vi "Save Recall List Program.vi"(8 "error in (no error)":errorcluster, 9 "List Number (1)":u32=1 min=1 max=10 format="%#_0f", 10 "Save Recall List File (0:Save)":u16(ring) items=["Save", "Recall"], 11 "VISA resource name":refnum<visa-resource-name>) -> (0 "error out":errorcluster, 3 "VISA resource name out":refnum<visa-resource-name>)   [LabVIEW 2020, in "BK Precision 911X Series.lvlib"]
doc: "Saves or recalls list programs to or from internal memory of the instrument. When using this vi to save a list program, all list parameters and configurations will be saved to the location specified by <b>List File Number</b> in <b>Configure List Parameters.vi</b>.\nBefore saving a list program, run the <b>Configure List Parameters.vi</b> and <b>Configure List Sequence Repeat.vi</b> first and in order.\n\n<b>Note: List program functionality is not available on model 9117.</b>"
uses:
  BK Precision 911X Series.lvlib
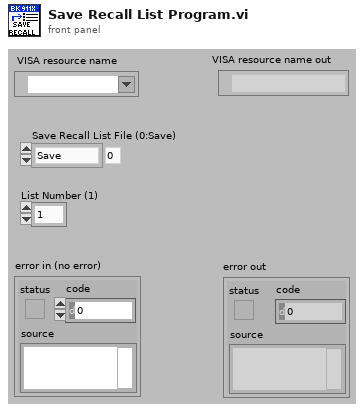
[diagram p1: front panel]
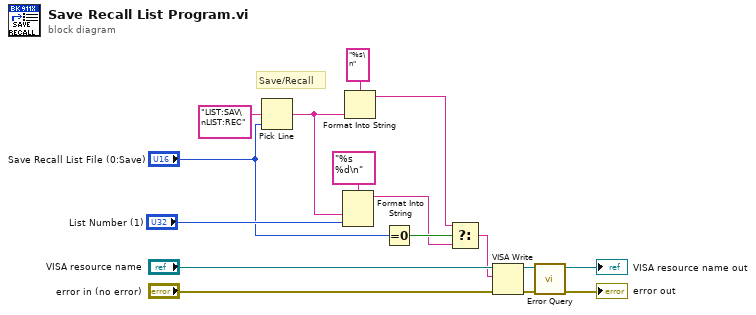
[diagram p0: block diagram]
diagram:
  # "Save/Recall"
  n1 = Pick Line(multi-line string="LIST:SAV\nLIST:REC", line index="Save Recall List File (0:Save)") -> (output string=w1:string)  [unwired: 1 in]
  n2 = Format Into String(format string="%s %d\n", w1, "List Number (1)") -> (resulting string=w5:string)  [unwired: 2 in, 1 out]
  n3 = Format Into String(format string="%s\n", w1) -> (resulting string=w3:string)  [unwired: 2 in, 1 out]
  n4 = Equal To 0?(x="Save Recall List File (0:Save)") -> (x = 0?=w7:bool)
  n5 = Select(t=w3, s=w7, f=w5) -> (s? t:f=w2:string)
  n6 = VISA Write(VISA resource name="VISA resource name", write buffer=w2, error in (no error)="error in (no error)") -> (VISA resource name out=w16:refnum<visa-resource-name>, error out=w15:errorcluster)  [unwired: 1 out]
  n7 = call "Error Query.vi"("error in (no error)"=w15, "VISA resource name"=w16) -> ("error out"=→"error out":errorcluster, "VISA resource name out"=→"VISA resource name out":refnum<visa-resource-name>)  [unwired: 6 in, 2 out]
